vi "ReadMultiDriveCounters.vi"(0 "Recheck if Moved?":bool, 1 "Matched Configurations":T1[](array[typedef]) {"Static Drive Configuration"."Indexer Mode  (FSA)" items=["Incremental", "Absolute"]; "Static Drive Configuration"."Buffer at Stop (SSH)" items=["Clear buffer", "Save and Continue"]; "Static Drive Configuration"."Buffer at Limit (SSG)" items=["Clear buffer", "Save and Continue"]; "Static Drive Configuration"."RS232 Echo Control (SSA)" items=["Echo ON", "Echo OFF"]; "Static Drive Configuration"."Reference edge of Home (OSH)" items=["CW", "CCW"]; "Static Drive Configuration"."Encoder Z for Home (OSD)" items=["Don't use", "Enable"]; "Static Drive Configuration"."Home Switch Sense (OSC)" items=["Normally Open", "Normally Closed"]; "Static Drive Configuration"."Home Position (OSB)" items=["Anywhere in Switch", "Edge of Switch"]; "Static Drive Configuration"."Limit Switch Sense (OSA)" items=["Normally Closed", "Normally Open"]; "Static Drive Configuration"."Limit Disable (LD)" items=["Both Enabled", "CW Disabled", "CCW Disabled", "Both Disabled"]; "Static Drive Configuration"."Stall Detect (FSH)" items=["Disable", "Enable"]; "Static Drive Configuration"."OP2 in Deadband (FSG)" items=["Don't Use", "ACTIVATE"]; "Static Drive Configuration"."Stop on Trigger 3 (FSF)" items=["Ignore", "STOP!"]; "Static Drive Configuration"."Activate OP1 on stall (FSE)" items=["Do not Activate", "ACTIVATE!"]; "Static Drive Configuration"."Stop on Stall (FSD)" items=["Continue", "STOP"]; "Static Drive Configuration"."Position Maintenance (FSC)" items=["Disabled", "Enabled"]; "Static Drive Configuration"."Step Mode  (FSB)" items=["Motor", "Encoder"]; "Static Drive Configuration"."Encoder Resolution (ER)" min=1 max=50000; "Static Drive Configuration"."Dead Band Window (DW)" min=0 max=999999999; "Static Drive Configuration"."Dead Band (DB)" min=0 max=999999999; "Static Drive Configuration"."Correction Gain % (CG)" items=["n/a", "12.5", "25", "37.5", "50", "62.5", "75", "87.5", "100"]; "Channel Properties"."Current Pos" format="%.2f"; "Channel Properties"."Backlash/Eng units" format="%.2f"; "Channel Properties"."Pulses/rev" format="%.2f"; "Channel Properties"."Pos Tolerance" format="%.2f"; "Channel Properties"."Pulses/unit" format="%.2f"; "Channel Properties"."Acc. Min" format="%.2f"; "Channel Properties"."Acc. Max" format="%.2f"; "Channel Properties"."Vel. Min" format="%.2f"; "Channel Properties"."Vel. Max" format="%.2f"; "Channel Properties"."Acc. Default" format="%.2f"; "Channel Properties"."Vel. Default" format="%.2f"}) -> (2 "Pulses":dbl[](array[numeric]), 3 "Eng units":dbl[](array[numeric]) format="%.2f", 4 "Error String":string)   [LabVIEW 2010]
uses:
  AxisConfigCluster.ctl
  DriveProperties.ctl
  DriveStaticConfig.ctl
  GenericDriveCommand.ctl
  Anemometry/Anemometry Sub Vis/Controls/In_Range.ctl
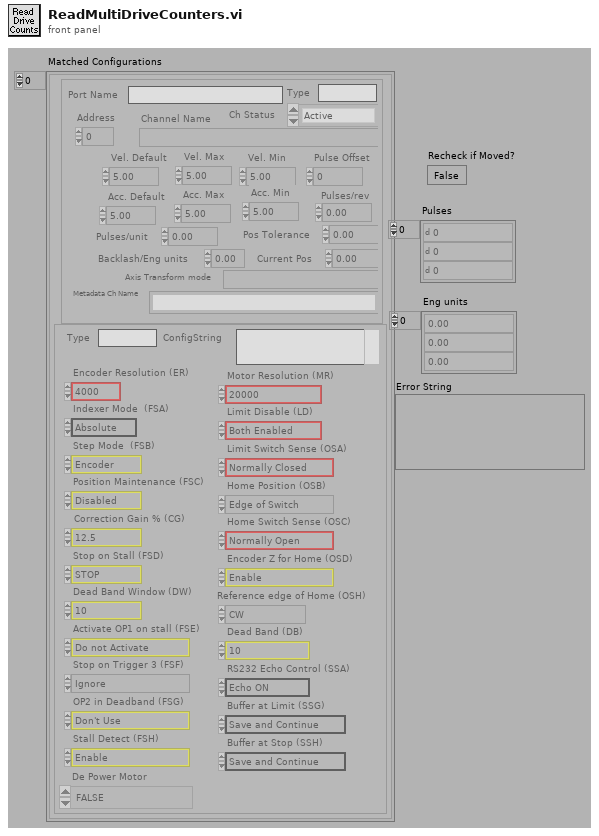
[diagram p1: front panel]
types:
  T1 = typedef "AxisConfigCluster.ctl" = cluster{"Channel Properties":T2, "Static Drive Configuration":T3}
  T2 = typedef "DriveProperties.ctl" = cluster{"Channel Name":string, "Vel. Default":dbl, "Acc. Default":dbl, "Vel. Max":dbl, "Vel. Min":dbl, "Acc. Max":dbl, "Acc. Min":dbl, "Pulses/unit":dbl, "Address":u8, "Pulse Offset":i32, "Pos Tolerance":dbl, "Pulses/rev":dbl, "Backlash/Eng units":dbl, "Current Pos":dbl, "Ch Status":enum16{"Active", "Offline", "Simulate"}, "Port Name":string, "Axis Transform mode":string, "Metadata Ch Name":string, "Type":string}
  T3 = typedef "DriveStaticConfig.ctl" = cluster{"Correction Gain % (CG)":u16, "Dead Band (DB)":i32, "Dead Band Window (DW)":i32, "Encoder Resolution (ER)":i32, "Step Mode  (FSB)":u16, "Position Maintenance (FSC)":u16, "Stop on Stall (FSD)":u16, "Activate OP1 on stall (FSE)":u16, "Stop on Trigger 3 (FSF)":u16, "OP2 in Deadband (FSG)":u16, "Stall Detect (FSH)":u16, "Limit Disable (LD)":u16, "Motor Resolution (MR)":enum16{"200", "400", "1000", "2000", "4000", "5000", "10000", "12800", "18000", "20000", "21600", "25000", "25400", "25600", "36000", "50000", "278528", "425984", "507904", "614400", "655360", "819200", "1024000"}, "Limit Switch Sense (OSA)":u16, "Home Position (OSB)":u16, "Home Switch Sense (OSC)":u16, "Encoder Z for Home (OSD)":u16, "Reference edge of Home (OSH)":u16, "RS232 Echo Control (SSA)":u16, "Buffer at Limit (SSG)":u16, "Buffer at Stop (SSH)":u16, "Indexer Mode  (FSA)":u16, "Type":string, "ConfigString":string, "De Power Motor":enum16{"TRUE", "FALSE"}}
  T4 = typedef "In_Range.ctl" = enum16{"%", "±", "% & ±"}
  T5 = typedef "GenericDriveCommand.ctl" = string
  T6 = enum16{"A-    Acceleration (rps)", "B-    Buffer Status", "C-    Continue", "CG-  Correction Gain", "CR-  Cariage Return", "D-    Distance (pulses)", "DB-  Dead Band (encoder steps)", "DW- Deadband Window (encoder steps)", "E-    Enable Communications", "ER-  Encoder Resolution (steps/rev)", "F-    Disable Communications", "FS-  Encoder Functions Report", "FSA- Incremental/Absolute (0/1)", "FSB- Motor/Encoder Step Mode (0/1)", "FSC- Enable/Disable Position Maint. (1/0)", "FSD- Stop/Continue on Stall (1/0)", "FSE- Activate o/p1 on Stall (1/0)", "FSF- Stop Motion on Trig3 (1/0)", "FSG- Activate o/p2 in Deadband (1/0)", "FSH- Enable Stall Detect (1/0)", "G- Go", "GH- Go Home and Zero (+/-V)", "^H- Delete ", "H- Direction Reverse/CCW/CW (0,1,2)", "IS- Input Status", "K- Kill", "L- Loop (n)", "LD- Limit DISABLE (0-none,1-CW,2-CCW,3-Both)", "LF- Line Feed", "MC- Mode Continuous", "MN- Mode Normal", "MPA- Motor Postion Absolute", "MPI- Motor Position Incremental", "MR- Motor Resolution (Drive Steps/rev)", "N- End of Loop", "O- Output (00,01,10,11)", "OS- Report Homing Setup", "OSA- NO/NC Limits (1/0)", "OSB- Back Up to Home/Edge? (0/1)", "OSC- NO/NC Home Switch (1/0)", "OSD- Enable Encoder Z for Home (0/1)", "OSH- Reference Edge for Home CW/CCW (0/1)", "PR- Report ABSOLUTE Position", "PS- Pause until Continue", "PX- Report Absolute ENCODER Position", "PZ- Zero Absolute Counter", "\"- Quote (17 ASCII +Space)", "Q- Enter/Exit Velocity Profiling (1/0)", "R- Request Indexer Status", "RA- Report Limit Switch Status", "RB- Report Loop, Pause, Shutdown, Trigger Status", "RC- Report Closed Loop Status", "RM- Velocity Streaming Rate Multiplier (000-FFF)", "RV- Report Revision Level", "S- Controlled Stop", "SN- Debounce (1-1000ms)", "SS- Report Software Switch Status", "SSA- Disable RS232 Echo (1/0)", "SSG- Clear/Save Command Buffer on Limit (0/1)", "SSH- Clear/Save Command Buffer on Stop (0/1)", "ST- Shutdown (1/0)", "SV- Servoing Setting (0,1,2,3)", "T- Time Delay (0.01-99999.99)", "TR- Wait for Trigger High/Low/Ignore (1/0/X)", "TS- Report Trigger Status", "U- Pause after Move Until Continue", "V- Velocity (0.01-50.00 revs/sec)", "W1- Report Relative Position <Signed Binary>", "W3- Report Relative Position <Hexadecimal>", "Y- Abort Loop at N", "Z-    Reset to Defaults", "#-    Disable/Set Soft Addresses (0/1-255)"}
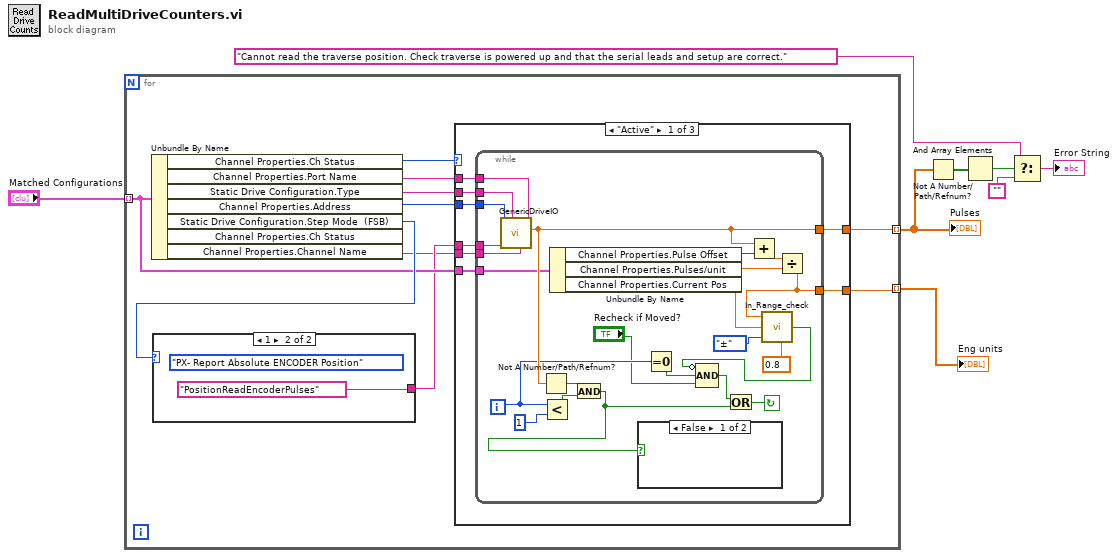
[diagram p0: block diagram]
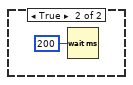
[diagram p2: hidden frame]
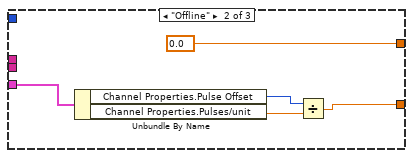
[diagram p3: hidden frame]
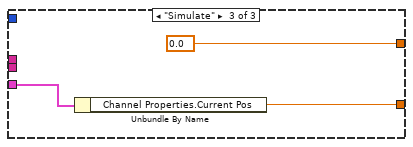
[diagram p4: hidden frame]
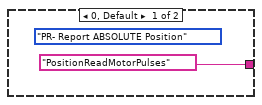
[diagram p5: hidden frame]
diagram:
  n1 = for {
    tunnel: [w18] -> w6 mode=indexing
    tunnel: "Matched Configurations" -> [w14] mode=indexing
    tunnel: [w13] -> w7 mode=indexing
    n2 = Unbundle By Name(w14) -> ("Channel Properties.Ch Status"=w11:enum16{"Active", "Offline", "Simulate"}, "Channel Properties.Port Name"=w15:string, "Static Drive Configuration.Type"=w10:string, "Channel Properties.Address"=w16:u8, "Static Drive Configuration.Step Mode  (FSB)"=w17:u16, "Channel Properties.Channel Name"=w9:string)  [unwired: 1 out]
    n3 = case shown="1" w17 {
      tunnel: [T5 "PositionReadMotorPulses" ("GenericDriveCommand") T5 "PositionReadEncoderPulses" ("GenericDriveCommand")] -> w12
      frame 0, Default {
        (unwired) T6."PR- Report ABSOLUTE Position" ("COMMAND")
      }
      frame 1 {
        (unwired) T6."PX- Report Absolute ENCODER Position" ("COMMAND")
      }
    }
    n4 = case shown="\"Active\"" w11 {
      tunnel: w12 -> [w26 _ _]
      tunnel: w16 -> [w25 _ _]
      tunnel: [w24 0.0 ("Numeric Reply") 0.0 ("Numeric Reply")] -> w18
      tunnel: w10 -> [w23 _ _]
      tunnel: w15 -> [w22 _ _]
      tunnel: w14 -> [w21 w56 w59]
      tunnel: [w20 w52 w57] -> w13
      tunnel: w9 -> [w19 _ _]
      frame "Active" {
        n5 = while {
          tunnel: [w38] -> w20
          tunnel: w21 -> [w40]
          tunnel: w22 -> [w48]
          tunnel: w23 -> [w28]
          tunnel: [w41] -> w24
          tunnel: w25 -> [w49]
          tunnel: w26 -> [w50]
          tunnel: w19 -> [w27]
          i -> [w35]
          stop <- w30 continue-if-true
          n6 = call "GenericDriveIO.vi"("GenericDriveCommand"=w50, "Channel Name"=w27, "Address"=w49, "Type"=w28, "Port Name"=w48) -> ("Numeric Reply"=w41:dbl)  [unwired: 1 in, 5 out]
          n7 = Not A Number/Path/Refnum?(number/path/refnum=w41) -> (NaN/Path/Refnum?=w46:bool)
          n8 = Less?(x=w35, y=1) -> (x < y?=w47:bool)
          n9 = Unbundle By Name(w40) -> ("Channel Properties.Pulse Offset"=w43:i32, "Channel Properties.Pulses/unit"=w44:dbl, "Channel Properties.Current Pos"=w39:dbl)
          n10 = And(x=w46, y=w47) -> (x .and. y?=w31:bool)
          n11 = case shown="False" w31 {
            frame False {
            }
            frame True {
              n12 = Wait (ms)(milliseconds to wait=u32 200) -> ()  [unwired: 1 out]
            }
          }
          n13 = Equal To 0?(x=w35) -> (x = 0?=w33:bool)
          n14 = Add(x=w41, y=w43) -> (x+y=w42:dbl)
          n15 = Divide(x=w42, y=w44) -> (x/y=w38:dbl)
          n16 = call "In_Range_check.vi"("±"=0.8, "Mode"=In_Range."±", "Value"=w39, "Setpoint"=w38) -> ("In Range"=w34:bool)  [unwired: 1 in, 2 out]
          n17 = Compound Arithmetic op=AND(invert w34, w33, "Recheck if Moved?") -> (w32:bool)
          n18 = Or(x=w32, y=w31) -> (x .or. y?=w30:bool)
        }
      }
      frame "Offline" {
        n19 = Unbundle By Name(w56) -> ("Channel Properties.Pulse Offset"=w54:i32, "Channel Properties.Pulses/unit"=w53:dbl)
        n20 = Divide(x=w54, y=w53) -> (x/y=w52:dbl)
      }
      frame "Simulate" {
        n21 = Unbundle By Name(w59) -> ("Channel Properties.Current Pos"=w57:dbl)
      }
    }
  }
  "Pulses" <- w6
  "Eng units" <- w7
  n22 = Not A Number/Path/Refnum?(number/path/refnum=w6) -> (NaN/Path/Refnum?=w5:bool[])
  n23 = And Array Elements(Boolean array=w5) -> (logical AND=w4:bool)
  n24 = Select(t="Cannot read the traverse position. Check traverse is powered up and that the serial leads and setup are correct.", s=w4, f="") -> (s? t:f=→"Error String":string)
